vi "Main.vi"(11 "Module Admin":refnum<class "Delacor_lib_QMH_Module Admin.lvclass">) -> ()   [LabVIEW 2021, in "Business Logic.lvlib"]
doc: "This template is based off of the Queued Message Handler design pattern and the Queued Message Handler project template that ships with LabVIEW.\n\nThe main difference is that the queue is private to this module and communication between modules is performed via Broadcast and Request events.\n\nRequest events are wrapped in public API methods and are handled in the Event Handling Loop (EHL) of this VI. Any module can register for Broadcast events sent by this module. The EHL generates messages based on user interface actions.\n\nThe Message Handling Loop (MHL) processes messages generated by the EHL, or by other messages. The messages are string values, so new messages can be added easily to the Message Cases case structure in the MHL. Each message cluster can also provide an optional value for Message Data, which is a variant that can be converted to whatever message-specific data is required.\n_____\nBased on DQMH Project Template 7.0.1.1316."
uses:
  Business Logic.lvlib
  <vilib>/Delacor/Delacor QMH/Libraries/Module Admin_class/Delacor_lib_QMH_Module Admin.lvclass
  Module Data--cluster.ctl
  <vilib>/Delacor/Delacor QMH/Libraries/Message Queue_class/Delacor_lib_QMH_Message Queue.lvclass/Delacor_lib_QMH_Message Queue.ctl
  Stop Argument--cluster.ctl
  <vilib>/Delacor/Delacor QMH/Libraries/Module Admin_class/Delacor_lib_QMH_Module Admin.lvclass/Delacor_lib_QMH_Module Admin.ctl
  <vilib>/Utility/miscctls.llb/LVPointTypeDef.ctl
  <vilib>/Delacor/Delacor QMH/Libraries/Message Queue_class/Delacor_lib_QMH_Enqueue Message (Single).vi
  <vilib>/Delacor/Delacor QMH/Libraries/Module Admin_class/Delacor_lib_QMH_Get External Launch.vi
  <vilib>/Delacor/Delacor QMH/Libraries/Message Queue_class/Delacor_lib_QMH_Message Queue.lvclass
  Signal Generator/Signal Generator.lvlib
  Log/Log.lvlib
  UI/UI.lvlib
panel:
  out "error out":errorcluster
  out "Status":string
  in  "Simulate MHL Error":bool
  in  "Simulate EHL Error":bool
  # "Other processes communicate with this Module via its Public API (wrappers for its Request Events).\n\nThis Module communicates with other processes via its Broadcast Events.\nAny process that wants to receive these messages can register for this module's Broadcast events."
  # "This template is for the DQMH framework. See the block diagram for more information on how to use this template."
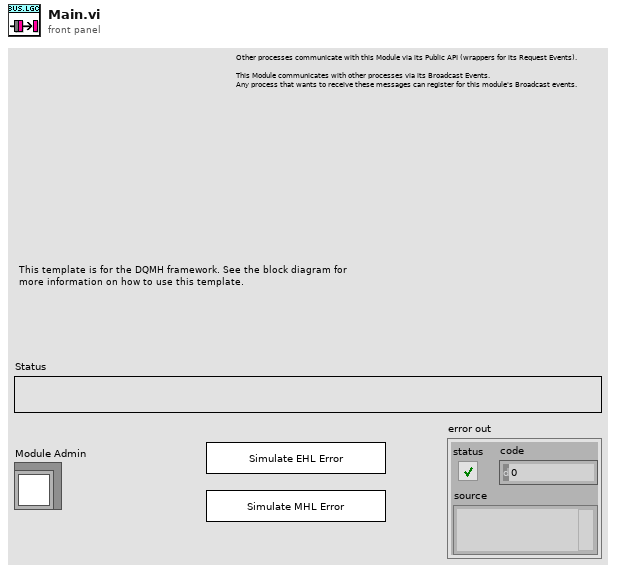
[diagram p1: front panel]
types:
  T1 = typedef "Business Logic.lvlib/Request Events--cluster.ctl" = cluster{"Stop Module":refnum<user-event>, "Show Panel":refnum<user-event>, "Hide Panel":refnum<user-event>, "Get Module Execution Status":refnum<user-event>, "Show Diagram":refnum<user-event>}
  T2 = typedef "Signal Generator.lvlib/Broadcast Events--cluster.ctl" = cluster{"Module Did Init":refnum<user-event>, "Status Updated":refnum<user-event>, "Error Reported":refnum<user-event>, "Module Did Stop":refnum<user-event>, "Update Module Execution Status":refnum<user-event>, "Signal Updated":refnum<user-event>}
  T3 = typedef "Log.lvlib/Broadcast Events--cluster.ctl" = cluster{"Module Did Init":refnum<user-event>, "Status Updated":refnum<user-event>, "Error Reported":refnum<user-event>, "Module Did Stop":refnum<user-event>, "Update Module Execution Status":refnum<user-event>}
  T4 = typedef "UI.lvlib/Broadcast Events--cluster.ctl" = cluster{"Module Did Init":refnum<user-event>, "Status Updated":refnum<user-event>, "Error Reported":refnum<user-event>, "Module Did Stop":refnum<user-event>, "Update Module Execution Status":refnum<user-event>, "Record Button Pressed":refnum<user-event>, "Signal Parameters Changed":refnum<user-event>}
  T5 = typedef "Business Logic.lvlib/Module Data--cluster.ctl" = cluster{"Status":string}
  T6 = enum32{"invalid lock state", "Not Locked", "Locked (No Password)", "Password-protected"}
  T7 = typedef "Business Logic.lvlib/Stop Argument--cluster.ctl" = cluster{"Origin":string, "Exit via Stop Module Req?":bool, "Wait for Module to stop?":bool}
  T8 = typedef "LVPointTypeDef.ctl" = cluster{"Horizontal":i16, "Vertical":i16}
  T9 = enum32{"Invalid", "Standard", "Closed", "Hidden", "Minimized", "Maximized"}
  T10 = enum16{"Sine Wave", "Triangle Wave", "Square Wave", "Sawtooth Wave"}
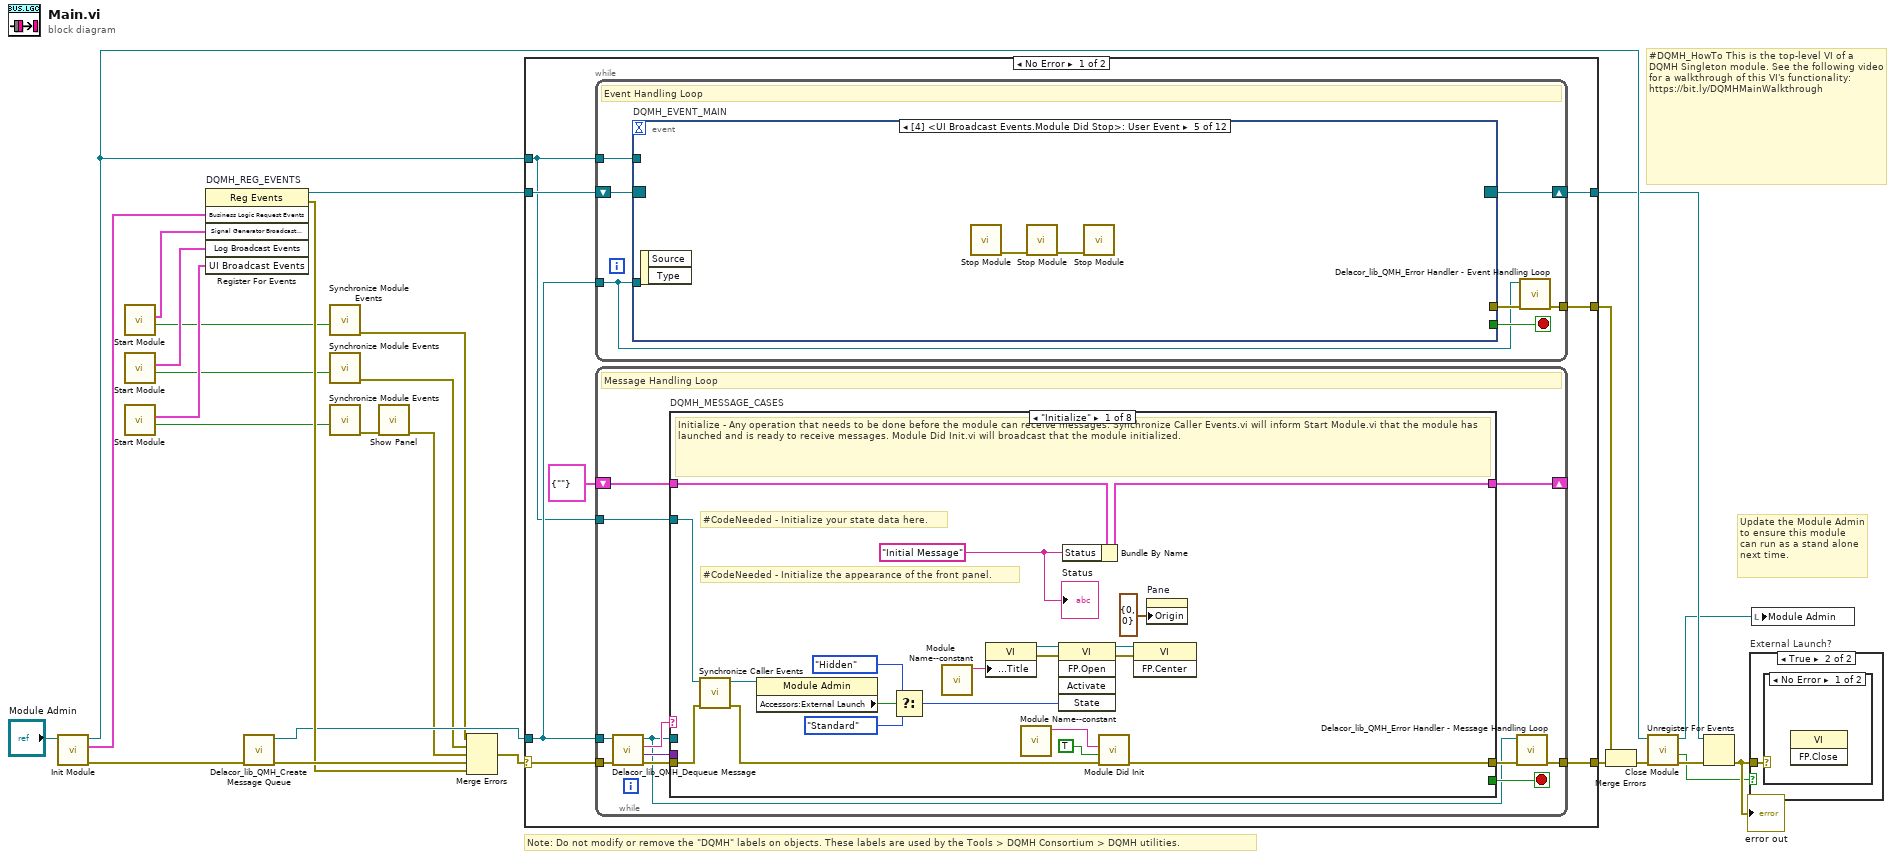
[diagram p0: block diagram]
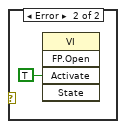
[diagram p3: hidden frame]
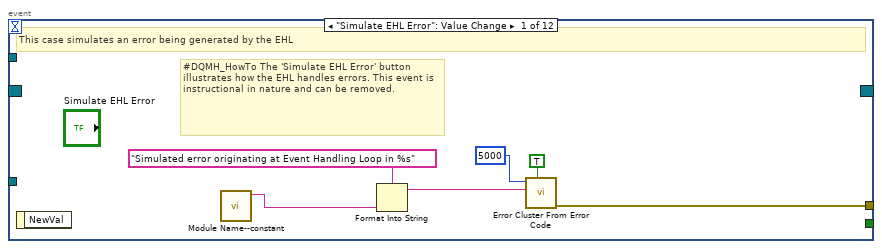
[diagram p4: hidden frame]
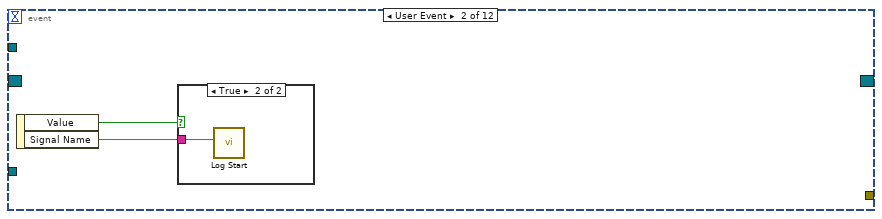
[diagram p5: hidden frame]
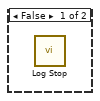
[diagram p6: hidden frame]
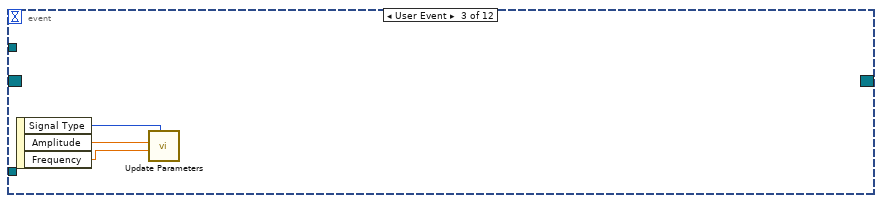
[diagram p7: hidden frame]
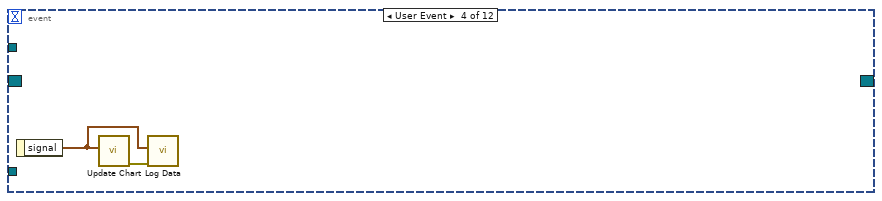
[diagram p8: hidden frame]
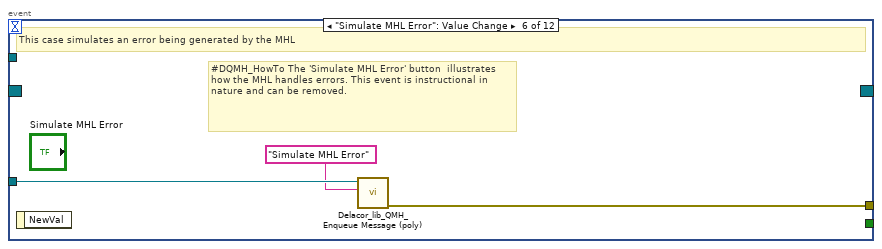
[diagram p9: hidden frame]
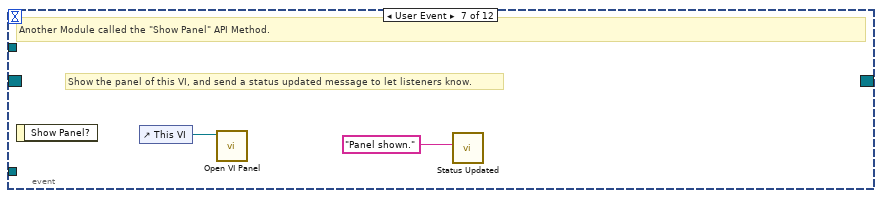
[diagram p10: hidden frame]
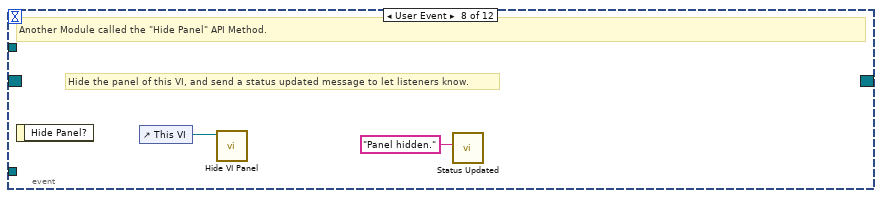
[diagram p11: hidden frame]
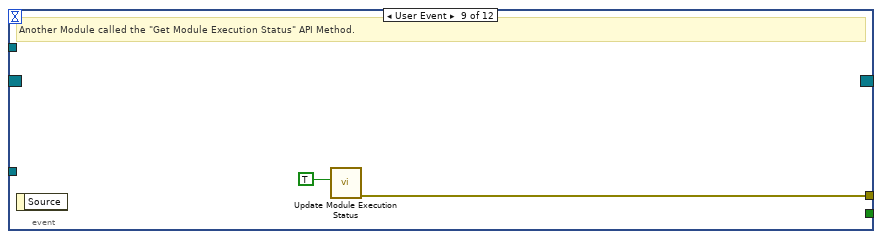
[diagram p12: hidden frame]
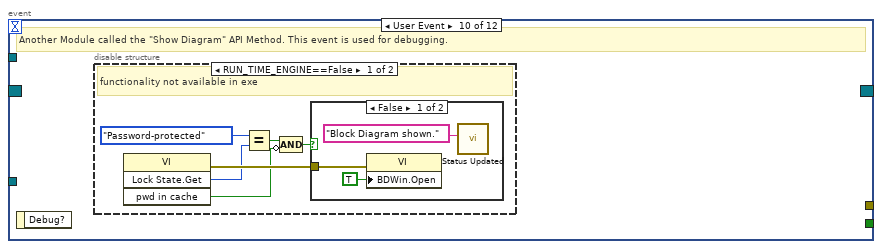
[diagram p13: hidden frame]
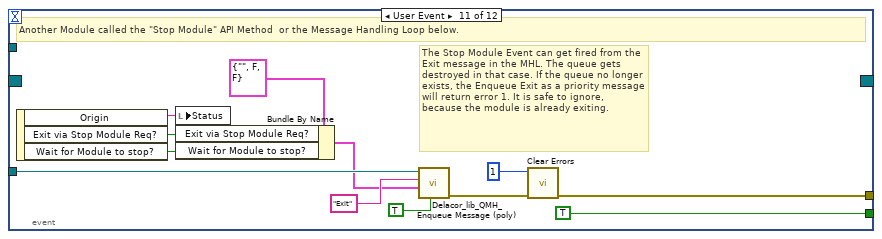
[diagram p16: hidden frame]
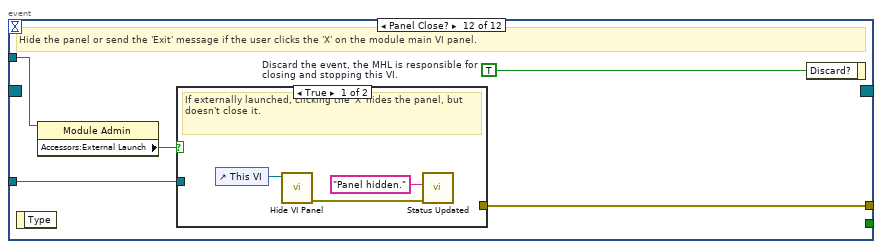
[diagram p17: hidden frame]
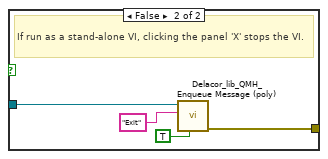
[diagram p18: hidden frame]
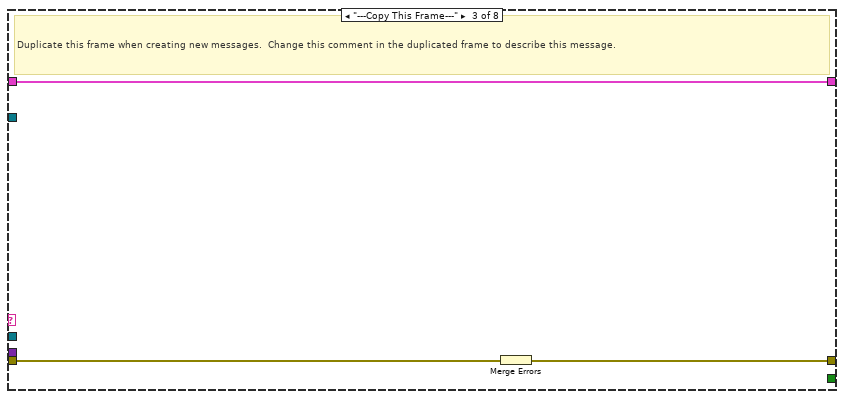
[diagram p20: hidden frame]
diagram:
  # "#DQMH_HowTo This is the top-level VI of a DQMH Singleton module. See the following video for a walkthrough of this VI's functionality: https://bit.ly/DQMHMainWalkthrough"
  # "Note: Do not modify or remove the \"DQMH\" labels on objects. These labels are used by the Tools > DQMH Consortium > DQMH utilities."
  # "Update the Module Admin to ensure this module can run as a stand alone next time."
  n1 = call "Init Module.vi"("Singleton Module Admin in"="Module Admin") -> ("error out"=w26:errorcluster, "Business Logic Request Events"=w15:T1, "Singleton Module Admin out"=w18:refnum<class "Delacor_lib_QMH_Module Admin.lvclass">)  [unwired: 8 in]
  n2 = call "Start Module.vi"() -> ("Wait for Event Sync?"=w7:bool, "Signal Generator Broadcast Events"=w10:T2)  [unwired: 8 in, 2 out]
  n3 = call "Start Module.vi"() -> ("Wait for Event Sync?"=w6:bool, "Log Broadcast Events"=w9:T3)  [unwired: 8 in, 2 out]
  n4 = call "Start Module.vi"() -> ("Wait for Event Sync?"=w5:bool, "UI Broadcast Events"=w8:T4)  [unwired: 8 in, 2 out]
  n5 = register-events "DQMH_REG_EVENTS"(w15, w10, w9, w8) -> (reference out=w16:refnum<event-registration>, error out=w19:errorcluster)  [unwired: 2 in]
  n6 = call <vilib>:"Delacor_lib_QMH_Create Message Queue.vi"("error in"=w26) -> ("error out"=w21:errorcluster, "Message Queue"=w14:refnum<class "Delacor_lib_QMH_Message Queue.lvclass">)  [unwired: 9 in]
  n7 = call "Synchronize Module Events.vi"("Wait for Event Sync?"=w7) -> ("error out"=w4:errorcluster)  [unwired: 10 in]
  n8 = call "Synchronize Module Events.vi"("Wait for Event Sync?"=w6) -> ("error out"=w3:errorcluster)  [unwired: 10 in]
  n9 = call "Synchronize Module Events.vi"("Wait for Event Sync?"=w5) -> ("error out"=w2:errorcluster)  [unwired: 10 in]
  n10 = call "Show Panel.vi"("error in"=w2) -> ("error out"=w1:errorcluster)  [unwired: 10 in]
  n11 = Merge Errors(w4, w3, w1, w21, w19) -> (w20:errorcluster)
  n12 = case shown="No Error" w20 {
    selector: w20 -> [w33 w198]
    tunnel: [w35 w197] -> w27
    tunnel: [w32 w196] -> w17
    tunnel: w16 -> [w30 w196]
    tunnel: w14 -> [w29 w191]
    tunnel: [w34 _] -> w24
    tunnel: w18 -> [w28 w192]
    frame No Error {
      n13 = while {
        tunnel: w29 -> [w36]
        shift-right: [w39] -> w32
        shift-left: w30 -> [w40]
        tunnel: [w41] -> w34
        tunnel: w28 -> [w37]
        stop <- w38 stop-if-true
        # "Event Handling Loop"
        n14 = event "DQMH_EVENT_MAIN" shown="[4] <UI Broadcast Events.Module Did Stop>: User Event" {
          selector: w40 -> [_ _ _ _ _ _ _ _ _ _ _ _]
          dyn-events: [_ _ _ _ _ _ _ _ _ _ _ _] -> w39
          timeout: _ -> [_ _ _ _ _ _ _ _ _ _ _ _]
          tunnel: [_ _ _ _ _ _ _ _ _ _ TRUE ("Discard?") _] -> w38
          tunnel: w36 -> [_ _ _ _ _ w60 _ _ _ _ w84 w91]
          tunnel: [w48 _ _ _ _ w61 _ _ w67 _ w87 w93] -> w42
          tunnel: w37 -> [_ _ _ _ _ _ _ _ _ _ _ w90]
          event "Simulate EHL Error": Value Change {
            # "#DQMH_HowTo The 'Simulate EHL Error' button  illustrates how the EHL handles errors. This event is instructional in nature and can be removed."
            # "This case simulates an error being generated by the EHL"
            n15 = event-data() -> ()  [unwired: 1 in, 1 out]
            n16 = call "Module Name--constant.vi"() -> ("Module Name"=w45:string)  [unwired: 11 in]
            n17 = Format Into String(format string="Simulated error originating at Event Handling Loop in %s", w45) -> (resulting string=w46:string)  [unwired: 2 in, 1 out]
            n18 = call <vilib>:"Error Cluster From Error Code.vi"("show call chain? (False)"=TRUE, "error message (\"\")"=w46, "error code (0)"=5000) -> ("error out"=w48:errorcluster)  [unwired: 6 in]
          }
          event User Event {
            n19 = event-data() -> ("Value"=w50:bool, "Signal Name"=w49:string)  [unwired: 1 in]
            n20 = case shown="True" w50 {
              tunnel: w49 -> [_ w51]
              frame False {
                n21 = call "Log Stop.vi"() -> ()  [unwired: 11 in, 1 out]
              }
              frame True {
                n22 = call "Log Start.vi"("Signal Name"=w51) -> ()  [unwired: 10 in, 1 out]
              }
            }
          }
          event User Event {
            n23 = event-data() -> ("Signal Type"=w54:T10, "Amplitude"=w53:dbl, "Frequency"=w52:dbl)  [unwired: 1 in]
            n24 = call "Update Parameters.vi"("signal type"=w54, "frequency"=w52, "amplitude"=w53) -> ()  [unwired: 8 in, 1 out]
          }
          event User Event {
            n25 = event-data() -> ("signal"=w55:waveform(dbl))  [unwired: 1 in]
            n26 = call "Update Chart.vi"("Signal"=w55) -> ("error out"=w56:errorcluster)  [unwired: 10 in]
            n27 = call "Log Data.vi"("error in"=w56, "Signal"=w55) -> ()  [unwired: 9 in, 1 out]
          }
          event User Event {
            n28 = event-data() -> ()  [unwired: 1 in, 2 out]
            n29 = call "Stop Module.vi"() -> ("error out"=w58:errorcluster)  [unwired: 11 in]
            n30 = call "Stop Module.vi"("error in"=w58) -> ("error out"=w57:errorcluster)  [unwired: 10 in]
            n31 = call "Stop Module.vi"("error in"=w57) -> ()  [unwired: 10 in, 1 out]
          }
          event "Simulate MHL Error": Value Change {
            # "#DQMH_HowTo The 'Simulate MHL Error' button  illustrates how the MHL handles errors. This event is instructional in nature and can be removed."
            # "This case simulates an error being generated by the MHL"
            n32 = event-data() -> ()  [unwired: 1 in, 1 out]
            n33 = call-poly <vilib>:"Delacor_lib_QMH_Enqueue Message (poly).vi"("Message"="Simulate MHL Error", "Message Queue in"=w60) -> ("error out"=w61:errorcluster)  [unwired: 8 in, 1 out]
          }
          event User Event {
            # "Show the panel of this VI, and send a status updated message to let listeners know."
            # "Another Module called the \"Show Panel\" API Method."
            n34 = event-data() -> ()  [unwired: 1 in, 1 out]
            n35 = control-ref of="This VI"() -> (w63:refnum<vi>)
            n36 = call "Open VI Panel.vi"("VI"=w63) -> ()  [unwired: 10 in, 1 out]
            n37 = call "Status Updated.vi"("Status"="Panel shown." ("format string")) -> ()  [unwired: 10 in, 1 out]
          }
          event User Event {
            # "Hide the panel of this VI, and send a status updated message to let listeners know."
            # "Another Module called the \"Hide Panel\" API Method."
            n38 = event-data() -> ()  [unwired: 1 in, 1 out]
            n39 = control-ref of="This VI"() -> (w65:refnum<vi>)
            n40 = call "Hide VI Panel.vi"("VI"=w65) -> ()  [unwired: 10 in, 1 out]
            n41 = call "Status Updated.vi"("Status"="Panel hidden." ("format string")) -> ()  [unwired: 10 in, 1 out]
          }
          event User Event {
            # "Another Module called the \"Get Module Execution Status\" API Method."
            n42 = event-data() -> ()  [unwired: 1 in, 1 out]
            n43 = call "Update Module Execution Status.vi"("Running?"=TRUE) -> ("error out"=w67:errorcluster)  [unwired: 10 in]
          }
          event User Event {
            # "Another Module called the \"Show Diagram\" API Method. This event is used for debugging."
            n44 = event-data() -> ()  [unwired: 1 in, 1 out]
            n45 = disable-structure shown="RUN_TIME_ENGINE==False" {
              frame condition #0 (active) {
                # "functionality not available in exe"
                n46 = invoke on="Invoke Node" class="VI" method="Lock State.Get"() -> (error out=w73:errorcluster, "Get Lock State"=w72:T6, "pwd in cache"=w69:bool)  [unwired: 4 in, 1 out]
                n47 = Equal?(x=T6."Password-protected", y=w72) -> (x = y?=w70:bool)
                n48 = Compound Arithmetic op=AND(w70, invert w69) -> (w68:bool)
                n49 = case shown="False" w68 {
                  tunnel: w73 -> [w76 _]
                  frame False {
                    n50 = property on="Property Node" class="VI"(error in=w76, "BDWin.Open"=TRUE ("Block Diagram Window:Open")) -> ()  [unwired: 1 in, 2 out]
                    n51 = call "Status Updated.vi"("Status"="Block Diagram shown." ("format string")) -> ()  [unwired: 10 in, 1 out]
                  }
                  frame True {
                    # "Password-protected VI, and the password is not in the cache. Do not show the diagram."
                  }
                }
              }
              frame condition #1 {
              }
            }
          }
          event User Event {
            # "The Stop Module Event can get fired from the Exit message in the MHL. The queue gets destroyed in that case. If the queue no longer exists, the Enqueue Exit as a priority message will return error 1. It is safe to ignore, because the module is already exiting."
            # "Another Module called the \"Stop Module\" API Method  or the Message Handling Loop below."
            n52 = event-data() -> ("Origin"=w83:string, "Exit via Stop Module Req?"=w79:bool, "Wait for Module to stop?"=w78:bool)  [unwired: 1 in]
            n53 = local write "Status"(w83) -> ()
            n54 = Bundle By Name(cluster=T7 {"Origin"="", "Exit via Stop Module Req?"=FALSE, "Wait for Module to stop?"=FALSE} ("Stop Argument"), "Exit via Stop Module Req?"=w79, "Wait for Module to stop?"=w78) -> (w77:T7)
            n55 = call-poly <vilib>:"Delacor_lib_QMH_Enqueue Message (poly).vi"("Priority Message? (F)"=TRUE, "Message Data"=w77, "Message"="Exit", "Message Queue in"=w84) -> ("error out"=w88:errorcluster)  [unwired: 6 in, 1 out]
            n56 = call <vilib>:"Clear Errors.vi"("error in (no error)"=w88, "specific error code to clear (0: all)"=1) -> ("error out"=w87:errorcluster)  [unwired: 4 in, 1 out]
          }
          event Panel Close? {
            w92 = TRUE  # Discard the event, the MHL is responsible for closing and stopping this VI.
            # "Hide the panel or send the 'Exit' message if the user clicks the 'X' on the module main VI panel."
            n57 = event-data() -> ()  [unwired: 1 in, 1 out]
            n58 = property on="Property Node" class="Module Admin"(reference=w90) -> ("Accessors:External Launch"=w89:bool)  [unwired: 1 in, 2 out]
            n59 = case shown="True" w89 {
              tunnel: w91 -> [_ w99]
              tunnel: [_ w100] -> w93
              frame True {
                # "If externally launched, clicking the 'X' hides the panel, but doesn't close it."
                n60 = control-ref of="This VI"() -> (w96:refnum<vi>)
                n61 = call "Hide VI Panel.vi"("VI"=w96) -> ("error out"=w94:errorcluster)  [unwired: 10 in]
                n62 = call "Status Updated.vi"("error in"=w94, "Status"="Panel hidden." ("format string")) -> ()  [unwired: 9 in, 1 out]
              }
              frame False {
                # "If run as a stand-alone VI, clicking the panel 'X' stops the VI."
                n63 = call-poly <vilib>:"Delacor_lib_QMH_Enqueue Message (poly).vi"("Priority Message? (F)"=TRUE, "Message"="Exit", "Message Queue in"=w99) -> ("error out"=w100:errorcluster)  [unwired: 7 in, 1 out]
              }
            }
            n64 = event-data ("Event Filter Node")("Discard?"=w92) -> ()  [unwired: 1 in, 1 out]
          }
        }
        n65 = call-dynamic "Delacor_lib_QMH_Error Handler - Event Handling Loop.vi"("error in"=w42, "Message Queue in"=w36) -> ("dup error in"=w41:errorcluster)  [unwired: 8 in, 1 out]
      }
      n66 = while {
        tunnel: w29 -> [w101]
        shift-right: [w109] -> _
        shift-left: T5 {"Status"=""} ("Data Cluster") -> [w110]
        tunnel: w33 -> [w112]
        tunnel: [w104] -> w35
        tunnel: w28 -> [w105]
        stop <- w108 stop-if-true
        # "Message Handling Loop"
        n67 = call-dynamic "Delacor_lib_QMH_Dequeue Message.vi"("error in"=w112, "Message Queue in"=w101) -> ("error out"=w111:errorcluster, "Message Data"=w106:variant, "Message"=w107:string, "Message Queue out"=w102:refnum<class "Delacor_lib_QMH_Message Queue.lvclass">)  [unwired: 6 in]
        n68 = case "DQMH_MESSAGE_CASES" shown="\"Initialize\"" w107 {
          selector: w107 -> [_ _ _ _ _ _ _ w186]
          tunnel: w102 -> [_ _ _ _ _ w152 w174 _]
          tunnel: w111 -> [w130 w134 w137 w139 w148 w159 w180 w189]
          tunnel: [w128 w134 w136 w139 w147 w155 w175 w190] -> w103
          tunnel: w110 -> [w119 w133 w135 w138 w145 w154 w173 w187]
          tunnel: [w118 w133 w135 w138 w145 w154 w173 w187] -> w109
          tunnel: [_ _ _ _ _ _ w172 _] -> w108
          tunnel: w106 -> [_ _ _ _ _ w153 w171 _]
          tunnel: w105 -> [w120 _ _ _ _ w151 w166 _]
          frame "Initialize" {
            w114 = "Initial Message" ("Initial Message")
            # "#CodeNeeded - Initialize the appearance of the front panel."
            # "#CodeNeeded - Initialize your state data here."
            # "Initialize - Any operation that needs to be done before the module can receive messages. Synchronize Caller Events.vi will inform Start Module.vi that the module has launched and is ready to receive messages. Module Did Init.vi will broadcast that the module initialized."
            n69 = call "Synchronize Caller Events.vi"("error in"=w130, "Singleton Module Admin in"=w120) -> ("error out"=w129:errorcluster, "Singleton Module Admin out"=w115:refnum<class "Delacor_lib_QMH_Module Admin.lvclass">)  [unwired: 8 in]
            n70 = property on="Property Node" class="Module Admin"(reference=w115) -> ("Accessors:External Launch"=w124:bool)  [unwired: 1 in, 2 out]
            n71 = Select(t=T9."Hidden" ("State"), s=w124, f=T9."Standard" ("State")) -> (s? t:f=w121:T9)
            n72 = call "Module Name--constant.vi"() -> ("Module Name"=w127:string)  [unwired: 11 in]
            n73 = property on="Property Node" class="VI"("Front Panel.Title"=w127) -> (reference out=w126:refnum<vi>, error out=w132:errorcluster)  [unwired: 2 in]
            n74 = call "Module Name--constant.vi"() -> ("Module Name"=w116:string)  [unwired: 11 in]
            n75 = invoke on="Invoke Node" class="VI" method="FP.Open"(reference=w126, error in=w132, "State"=w121) -> (reference out=w125:refnum<vi>, error out=w131:errorcluster)  [unwired: 2 in, 3 out]
            n76 = Bundle By Name(cluster=w119, "Status"=w114) -> (w118:T5)
            n77 = call "Module Did Init.vi"("error in"=w129, "Initialized?"=TRUE, "Origin"=w116) -> ("error out"=w128:errorcluster)  [unwired: 8 in]
            n78 = invoke on="Invoke Node" class="VI" method="FP.Center"(reference=w125, error in=w131) -> ()  [unwired: 1 in, 3 out]
            n79 = property on="Pane" class="Pane"("Origin"=T8 {"Horizontal"=0, "Vertical"=0}) -> ()  [unwired: 2 in, 2 out]
            "Status" <- w114
          }
          frame "---Module Specific---" {
            # "Separator -- The following cases handle messages specific to this Module."
          }
          frame "---Copy This Frame---" {
            # "Duplicate this frame when creating new messages.  Change this comment in the duplicated frame to describe this message."
            n80 = Merge Errors(w137) -> (w136:errorcluster)
          }
          frame "---Exit and Error Handling---" {
            # "Separator - The following cases handle errors and exit messages."
          }
          frame "Simulate MHL Error" {
            # "#DQMH_HowTo The 'Simulate MHL Error' button  illustrates how the MHL handles errors. This event is instructional in nature and can be removed."
            # "Simulate an error occurring at the MHL"
            n81 = call "Module Name--constant.vi"() -> ("Module Name"=w141:string)  [unwired: 11 in]
            n82 = Format Into String(format string="Simulated error originating at Message Handling Loop in %s", w141) -> (resulting string=w142:string)  [unwired: 2 in, 1 out]
            n83 = call <vilib>:"Error Cluster From Error Code.vi"("show call chain? (False)"=TRUE, "error message (\"\")"=w142, "error code (0)"=5001) -> ("error out"=w146:errorcluster)  [unwired: 6 in]
            n84 = Merge Errors(w148, w146) -> (w147:errorcluster)
          }
          frame "Error" {
            # "#CodeRecommended - If the module is running in standalone mode (External Launch = FALSE), this code will pop up an error dialog and call the 'Exit' message if an error occurs. Add more fine-grained error management here."
            # "Error - Check the error message data and respond accordingly. This message is sent by the \"Error Handler\" VIs at the end of each loop in this application."
            n85 = property on="Property Node" class="Module Admin"(reference=w151) -> ("Accessors:External Launch"=w150:bool)  [unwired: 1 in, 2 out]
            n86 = Variant To Data(error in=w159, type=errorcluster {"status"=FALSE, "code"=0, "source"=""} ("error constant"), Variant=w153) -> (data=w149:errorcluster, error out=w157:errorcluster)
            n87 = local write "error out"(w149) -> ()
            n88 = call "Error Reported.vi"("Error"=w149) -> ()  [unwired: 10 in, 1 out]
            n89 = case shown="False" w150 {
              tunnel: [w164 _] -> w156
              tunnel: w152 -> [w162 _]
              tunnel: w149 -> [w163 _]
              frame False {
                n90 = disable-structure shown="Default" {
                  disable-tunnel: w163 -> [w165 _]
                  frame condition #0 (active) {
                    # "If the module is running standalone, then pop up an error dialog and call the \"Exit\" message."
                    n91 = call <vilib>:"Simple Error Handler.vi"("error in (no error)"=w165) -> ()  [unwired: 4 in, 5 out]
                  }
                  frame condition #1 {
                    # "To prevent the Simple Error Handler VI from being loaded (e.g. when deploying to a Real-Time target), add the Conditional Disable Symbol \"DQMH_Disable_SEH\" to your project and set it to TRUE."
                  }
                }
                n92 = call-poly <vilib>:"Delacor_lib_QMH_Enqueue Message (poly).vi"("Priority Message? (F)"=TRUE, "Message"="Exit", "Message Queue in"=w162) -> ("error out"=w164:errorcluster)  [unwired: 7 in, 1 out]
              }
              frame True {
                # "If the module was launched externally, calling the Error Reported broadcast VI is the only action performed by the \"Error\" message. The module's caller can then process the error appropriately."
              }
            }
            n93 = Merge Errors(w157, w156) -> (w155:errorcluster)
          }
          frame "Exit" {
            w170 = 91  # 91: not all Exit messages will have an argument
            w172 = TRUE  # Stop the VI
            # "Release the message queue reference"
            # "#CodeNeeded - Add any required cleanup code here."
            # "Exit - Exit the application."
            n94 = Variant To Data(error in=w180, type=T7 {"Origin"="", "Exit via Stop Module Req?"=FALSE, "Wait for Module to stop?"=FALSE} ("Stop Argument"), Variant=w171) -> (data=w168:T7, error out=w177:errorcluster)
            n95 = call <vilib>:"Clear Errors.vi"("error in (no error)"=w177, "specific error code to clear (0: all)"=w170) -> ("error out"=w179:errorcluster)  [unwired: 4 in, 1 out]
            n96 = control-ref of="This VI"() -> (w167:refnum<vi>)
            n97 = call-dynamic "Delacor_lib_QMH_Release Message Queue.vi"("error in"=w179, "Message Queue"=w174) -> ("error out"=w178:errorcluster)  [unwired: 9 in]
            n98 = call "Handle Exit.vi"("Stop Argument"=w168, "Admin in"=w166, "VI reference"=w167) -> ("error out"=w176:errorcluster)  [unwired: 7 in, 1 out]
            n99 = Merge Errors(w178, w176) -> (w175:errorcluster)
            n100 = call "Error Reported.vi"("Error"=w175) -> ()  [unwired: 10 in, 1 out]
          }
          frame Default {
            # "'Default' case only runs if there is a message that isn't defined in any of the other cases.  Output a programming error."
            n101 = call "Module Name--constant.vi"() -> ("Module Name"=w185:string)  [unwired: 11 in]
            n102 = Format Into String(format string="The invalid message string \"%s\" was received in the Message Handling Loop for module \"%s\".", w186, w185) -> (resulting string=w181:string)  [unwired: 2 in, 1 out]
            n103 = call <vilib>:"Error Cluster From Error Code.vi"("show call chain? (False)"=TRUE, "error message (\"\")"=w181, "error code (0)"=1) -> ("error out"=w188:errorcluster)  [unwired: 6 in]
            n104 = Merge Errors(w189, w188) -> (w190:errorcluster)
          }
        }
        n105 = call-dynamic "Delacor_lib_QMH_Error Handler - Message Handling Loop.vi"("error in"=w103, "Message Queue in"=w102) -> ("dup error in"=w104:errorcluster)  [unwired: 8 in, 1 out]
      }
    }
    frame Error {
      # "Synchronize Caller Events.vi will inform Start Module.vi that the module has launched and will let the code calling Start Module.vi register for broadcasts and would permit the caller receive the broadcast that an error occurred at launch time."
      n106 = call-dynamic "Delacor_lib_QMH_Release Message Queue.vi"("error in"=w198, "Message Queue"=w191) -> ("error out"=w197:errorcluster)  [unwired: 9 in]
      n107 = call "Synchronize Caller Events.vi"("Singleton Module Admin in"=w192) -> ("error out"=w199:errorcluster)  [unwired: 9 in, 1 out]
      n108 = call "Module Name--constant.vi"() -> ("Module Name"=w195:string)  [unwired: 11 in]
      n109 = Format Into String(format string="An error occurred during initialization. %s is no longer running.", w195) -> (resulting string=w193:string)  [unwired: 2 in, 1 out]
      n110 = Merge Errors(w197, w199) -> (w200:errorcluster)
      n111 = call "Error Reported.vi"("Additional Information"=w193, "Error"=w200) -> ()  [unwired: 9 in, 1 out]
    }
  }
  n112 = Merge Errors(w24, w27) -> (w23:errorcluster)
  n113 = call "Close Module.vi"("error in"=w23, "Module Admin in"=w18) -> ("error out"=w25:errorcluster, "External Launch"=w11:bool, "Module Admin out"=w12:refnum<class "Delacor_lib_QMH_Module Admin.lvclass">)  [unwired: 7 in]
  n114 = Unregister For Events(event registration refnum=w17, error in=w25) -> (error out=w22:errorcluster)
  "error out" <- w22
  n115 = case "External Launch?" shown="True" w11 {
    tunnel: w22 -> [_ w201]
    frame False {
    }
    frame True {
      n116 = case shown="No Error" w201 {
        frame No Error {
          n117 = invoke on="Invoke Node" class="VI" method="FP.Close"() -> ()  [unwired: 3 in, 3 out]
        }
        frame Error {
          n118 = invoke on="Invoke Node" class="VI" method="FP.Open"("Activate"=TRUE ("Activate?")) -> ()  [unwired: 4 in, 5 out]
        }
      }
    }
  }
  n119 = local write "Module Admin"(w12) -> ()
